vi "Actor Core.vi"(8 "error in":errorcluster, 11 "XY WFRM Plot in":refnum<class "XY WFRM Plot.lvclass">) -> (0 "error out":errorcluster, 3 "Actor out":refnum<class "Actor.lvclass">)   [LabVIEW 2016, in "XY WFRM Plot.lvclass"]
doc: "Plots listed TDMS data files"
uses:
  XY WFRM Plot.lvclass
  C:/github/LabActor/Template Module/Template Module.lvclass
  C:/github/LabActor/Plots/Plot/Plot.lvclass
  C:/Program Files/National Instruments/LabVIEW 2016/vi.lib/ActorFramework/Actor/Actor.lvclass
  <vilib>/ActorFramework/Actor/Actor.lvclass
  Plot types.ctl
  XY WFRM Plot.lvclass/XY WFRM Plot.ctl
  Template Module/Template Module.lvclass/Template Module.ctl
  Plot/Plot.lvclass/Plot.ctl
  <vilib>/ActorFramework/Actor/Actor.lvclass/Actor.ctl
  <vilib>/ActorFramework/Message Enqueuer/Message Enqueuer.lvclass/Message Enqueuer.ctl
  XY WFRM Plot Messages/Set Plot Type Msg/Set Plot Type Msg.lvclass/Set Plot Type Msg.ctl
  Plot Messages/Write Files Msg/Write Files Msg.lvclass/Write Files Msg.ctl
  Plot Messages/Write Keep # of preceding files Msg/Write File history depth Msg.lvclass/Write File history depth Msg.ctl
  Template Module/Read stop event.vi
  Read Plot type.vi
  Plot/WriteFile history depth.vi
  <vilib>/ActorFramework/Message Enqueuer/Init from Existing Queue.vi
  <vilib>/ActorFramework/Message Enqueuer/Enqueue.vi
  XY WFRM Plot Messages/Set Plot Type Msg/Set Plot Type Msg.lvclass
  C:/Program Files/National Instruments/LabVIEW 2016/vi.lib/ActorFramework/Message/Message.lvclass
  Plot Messages/Replot Msg/Replot Msg.lvclass
  Plot Messages/Write Files Msg/Write Files Msg.lvclass
  <vilib>/ActorFramework/Stop Msg/Stop Msg.lvclass
  Plot Messages/Write Keep # of preceding files Msg/Write File history depth Msg.lvclass
  <vilib>/ActorFramework/Message Priority Queue/Priority Enqueue.vi
  Plot/Plot.lvclass
  <vilib>/ActorFramework/Message Enqueuer/Message Enqueuer.lvclass
panel:
  in  "File history depth":i32=2
  out "Waveform Plot":waveform(sgl)[](graph)
  in  "Y column(s)":i32[](listbox)=[1]
  in  "X column":i32(listbox)
  in  "File(s)":path[](array[path])
  out "XY Plot":cluster{"Y":sgl[], "Y":sgl[]}[](graph)
  in  "Plot type":enum32{"X-Y Plot", "Waveform Plot"}(tab)
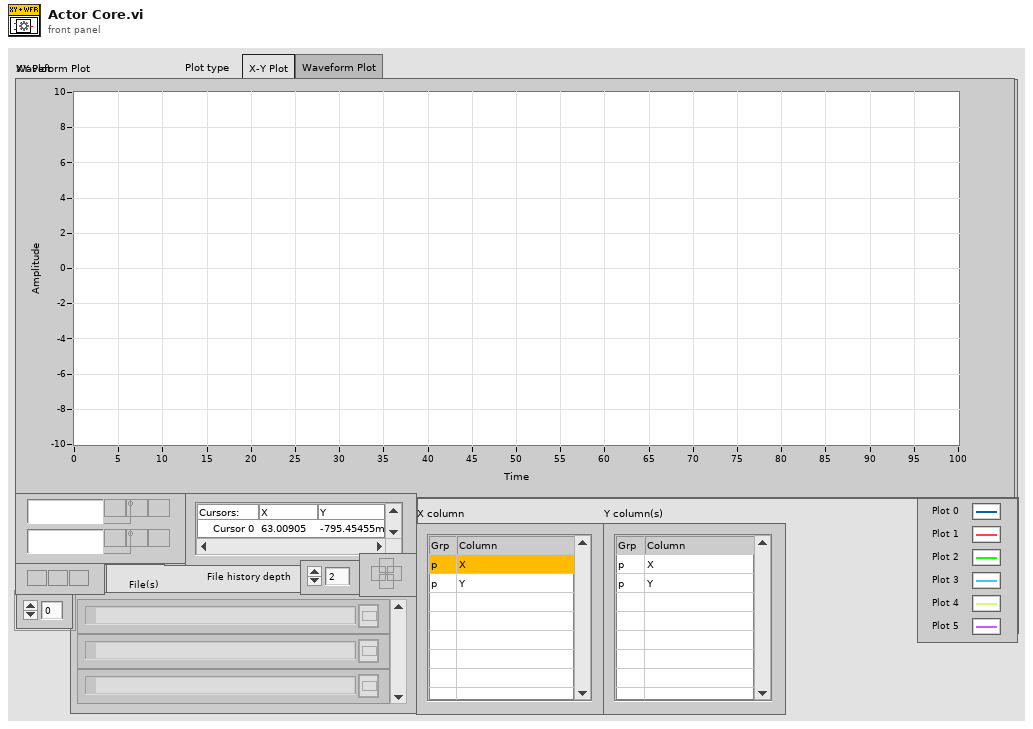
[diagram p1: front panel]
types:
  T1 = typedef "Plot types.ctl" = enum16{"Waveform Plot", "XY Plot", "Full XY"}
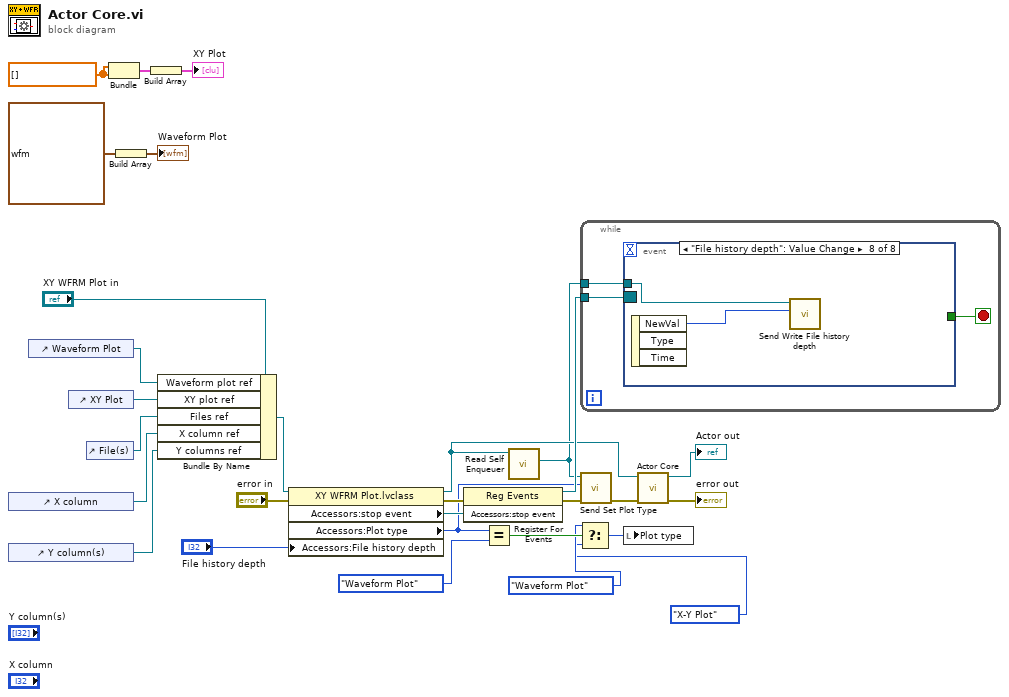
[diagram p0: block diagram]
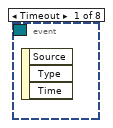
[diagram p2: hidden frame]
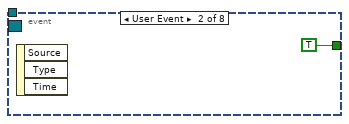
[diagram p3: hidden frame]
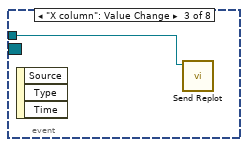
[diagram p4: hidden frame]
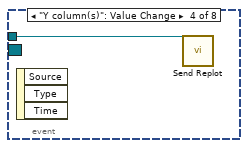
[diagram p5: hidden frame]
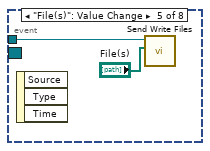
[diagram p6: hidden frame]
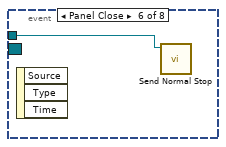
[diagram p7: hidden frame]
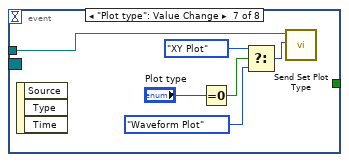
[diagram p8: hidden frame]
diagram:
  w16 = sgl[] [] ("Y")
  n1 = control-ref of="X column"() -> (w22:refnum<vi>)
  n2 = control-ref of="Y column(s)"() -> (w23:refnum<vi>)
  n3 = control-ref of="Waveform Plot"() -> (w12:refnum<vi>)
  n4 = control-ref of="XY Plot"() -> (w25:refnum<vi>)
  n5 = control-ref of="File(s)"() -> (w24:refnum<vi>)
  n6 = Bundle("Y"=w16, "Y"=w16) -> (w15:cluster{"Y":sgl[], "Y":sgl[]})  [unwired: 1 in]
  n7 = Build Array(waveform(sgl) {"t0"=timestamp(0 s since 1904-01-01), "dt"=1.0, "Y"=[]} ("Waveform")) -> (→"Waveform Plot":waveform(sgl)[])
  n8 = Build Array(w15) -> (→"XY Plot":cluster{"Y":sgl[], "Y":sgl[]}[])
  n9 = Bundle By Name(cluster="XY WFRM Plot in", "Waveform plot ref"=w12, "XY plot ref"=w25, "Files ref"=w24, "X column ref"=w22, "Y columns ref"=w23) -> (w26:refnum<class "XY WFRM Plot.lvclass">)
  n10 = property class="XY WFRM Plot.lvclass"(reference=w26, error in="error in", "Accessors:File history depth"="File history depth") -> (reference out=w13:refnum<class "XY WFRM Plot.lvclass">, error out=w19:errorcluster, "Accessors:stop event"=w21:refnum<user-event>, "Accessors:Plot type"=w5:T1)
  n11 = register-events(error in=w19, w21) -> (reference out=w20:refnum<event-registration>, error out=w9:errorcluster)  [unwired: 1 in]
  n12 = Equal?(x=w5, y=Plot_types."Waveform Plot" ("Plot type")) -> (x = y?=w10:bool)
  n13 = call <vilib>:"Read Self Enqueuer.vi"("Actor"=w13) -> ("Self Enqueuer"=w7:refnum<class "Message Enqueuer.lvclass">)  [unwired: 10 in]
  n14 = Select(t=enum32{"X-Y Plot", "Waveform Plot"}."Waveform Plot" ("Plot type"), s=w10, f=enum32{"X-Y Plot", "Waveform Plot"}."X-Y Plot" ("Plot type")) -> (s? t:f=w6:enum32{"X-Y Plot", "Waveform Plot"})
  n15 = while {
    tunnel: w20 -> [w32]
    tunnel: w7 -> [w30]
    stop <- w31 stop-if-true
    n16 = event shown="[7] \"File history depth\": Value Change" {
      selector: w32 -> [_ _ _ _ _ _ _ _]
      dyn-events: _ -> [_ _ _ _ _ _ _ _]
      timeout: _ -> [_ _ _ _ _ _ _ _]
      tunnel: [_ TRUE _ _ _ _ _ _] -> w31
      tunnel: w30 -> [_ _ w34 w35 w37 w38 w43 w46]
      event Timeout {
        n17 = event-data() -> ()  [unwired: 1 in, 3 out]
      }
      event User Event {
        n18 = event-data() -> ()  [unwired: 1 in, 3 out]
      }
      event "X column": Value Change {
        n19 = event-data() -> ()  [unwired: 1 in, 3 out]
        n20 = call "Send Replot.vi"("Message Enqueuer"=w34) -> ()  [unwired: 9 in, 2 out]
      }
      event "Y column(s)": Value Change {
        n21 = event-data() -> ()  [unwired: 1 in, 3 out]
        n22 = call "Send Replot.vi"("Message Enqueuer"=w35) -> ()  [unwired: 9 in, 2 out]
      }
      event "File(s)": Value Change {
        n23 = event-data() -> ()  [unwired: 1 in, 3 out]
        n24 = call "Send Write Files.vi"("Files"="File(s)", "Message Enqueuer"=w37) -> ()  [unwired: 8 in, 2 out]
      }
      event Panel Close {
        n25 = event-data() -> ()  [unwired: 1 in, 3 out]
        n26 = call <vilib>:"Send Normal Stop.vi"("Message Enqueuer"=w38) -> ()  [unwired: 10 in, 1 out]
      }
      event "Plot type": Value Change {
        n27 = event-data() -> ()  [unwired: 1 in, 3 out]
        n28 = Equal To 0?(x="Plot type") -> (x = 0?=w42:bool)
        n29 = Select(t=Plot_types."XY Plot" ("Plot type"), s=w42, f=Plot_types."Waveform Plot" ("Plot type")) -> (s? t:f=w41:T1)
        n30 = call "Send Set Plot Type.vi"("Plot type"=w41, "Message Enqueuer"=w43) -> ()  [unwired: 8 in, 2 out]
      }
      event "File history depth": Value Change {
        n31 = event-data() -> ("NewVal"=w45:i32)  [unwired: 1 in, 2 out]
        n32 = call "Send Write File history depth.vi"("File history depth"=w45, "Message Enqueuer"=w46) -> ()  [unwired: 8 in, 2 out]
      }
    }
  }
  n33 = call "Send Set Plot Type.vi"("error in (no error)"=w9, "Plot type"=w5, "Message Enqueuer"=w7) -> ("error out"=w8:errorcluster)  [unwired: 7 in, 1 out]
  n34 = local write "Plot type"(w6) -> ()
  n35 = call-parent "Actor Core.vi"("error in"=w8, "Measure Object in"=w13) -> ("error out"=→"error out":errorcluster, "Actor out"=→"Actor out":refnum<class "Actor.lvclass">)  [unwired: 8 in]
